vi "V004 - Final Labview.vi"() -> ()   [LabVIEW 2022 SP3]
uses:
  <vilib>/DAQmx/read.llb/DAQmx Read (Analog 1D DBL NChan 1Samp).vi
  <vilib>/DAQmx/create/channels.llb/DAQmx Create Channel (AI-Voltage-Basic).vi
  <vilib>/DAQmx/miscellaneous.llb/DAQmx Fill In Error Info.vi
panel:
  out "High Temperature":bool
  out "High Humidity":bool
  out "Fan Speed Chart":dbl(graph)
  out "Humidity Chart":dbl(graph)
  out "Temperature Chart":dbl(graph)
  in  "Turn Off":bool
  out "Speed 3":bool
  out "Humidity":dbl(knob) scale=0.0..100.0
  out "Temperature":dbl(knob) scale=0.0..40.0
  out "Speed 2":bool
  out "Speed 1":bool
  in  "Numeric Controller Sub":dbl format="%#_1g"
  out "Power On":bool
  in  "Power On":bool
  out "Connected":bool
  in  "VISA resource name":refnum<visa-resource-name>
  in  "Connect":bool
  in  "Numeric Controller Main":dbl
  # "SMART FAN"
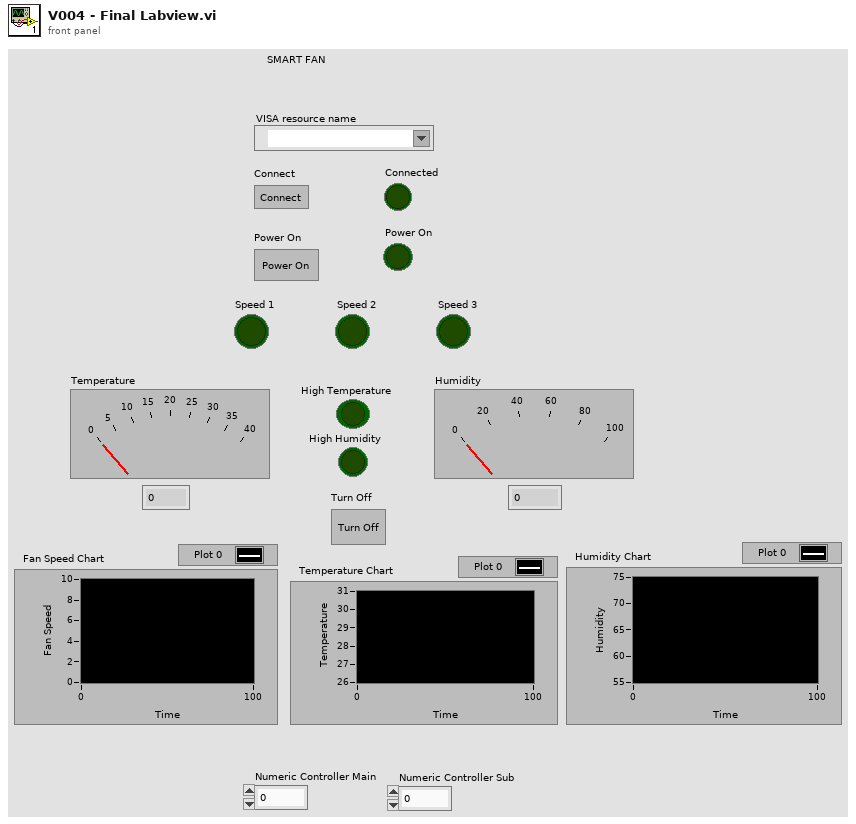
[diagram p1: front panel]
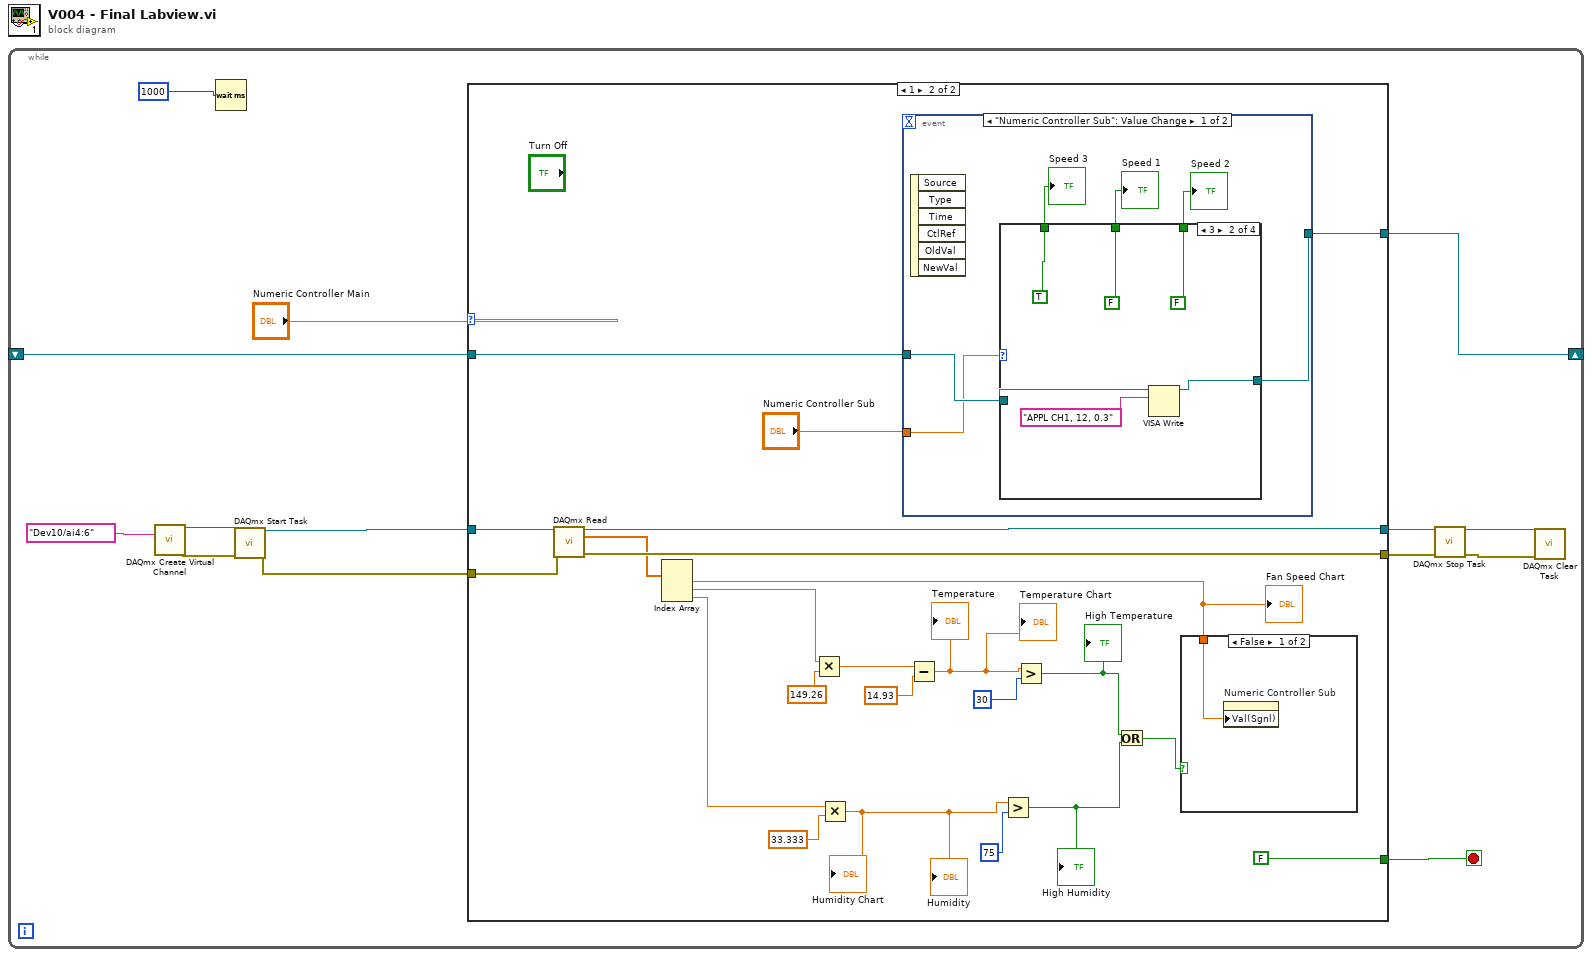
[diagram p0: block diagram]
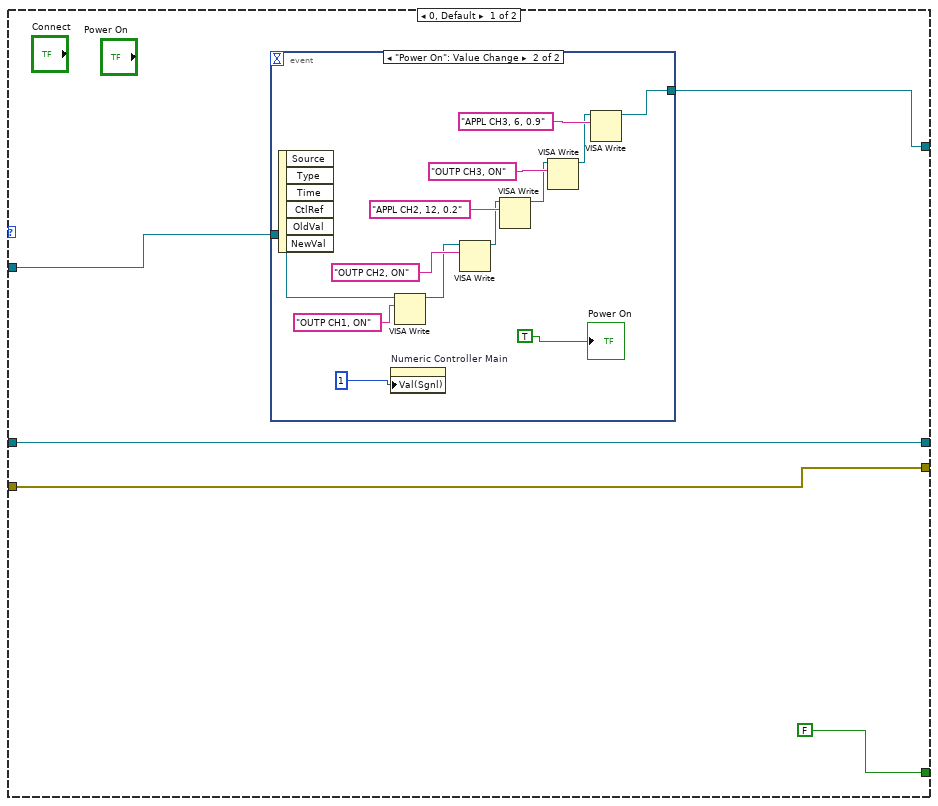
[diagram p2: hidden frame]
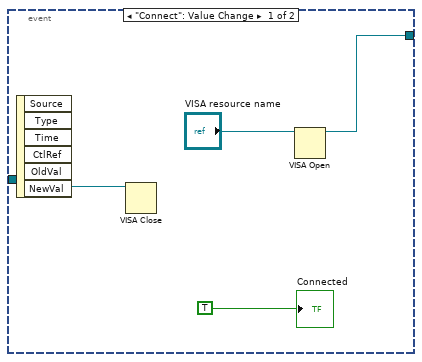
[diagram p3: hidden frame]
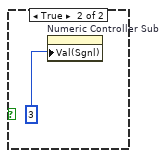
[diagram p4: hidden frame]
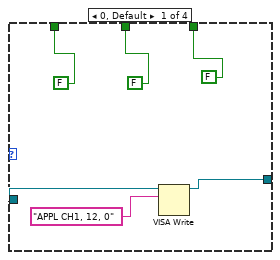
[diagram p5: hidden frame]
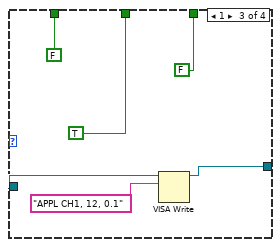
[diagram p6: hidden frame]
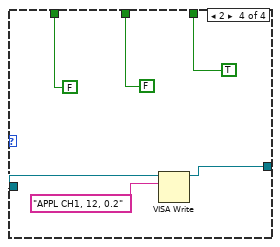
[diagram p7: hidden frame]
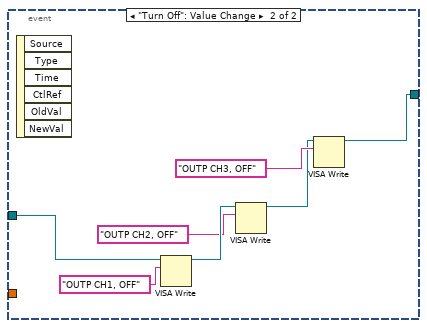
[diagram p8: hidden frame]
diagram:
  n1 = while {
    shift-right: [w13] -> _
    shift-left: _ -> [w14]
    stop <- w12 stop-if-true
    n2 = call-poly <vilib>:"DAQmx Create Virtual Channel.vi"("physical channels"=tag "Dev10/ai4:6") -> ("task out"=w10:refnum<k21>, "error out"=w6:errorcluster)  [unwired: 13 in]
    n3 = Wait (ms)(milliseconds to wait=1000) -> ()  [unwired: 1 out]
    n4 = call <vilib>:"DAQmx Start Task.vi"("task/channels in"=w10, "error in"=w6) -> ("task out"=w8:refnum<k21>, "error out"=w7:errorcluster)  [unwired: 12 in]
    n5 = case shown="1" "Numeric Controller Main" {
      tunnel: w14 -> [w19 w57]
      tunnel: [w18 w58] -> w13
      tunnel: [FALSE FALSE] -> w12
      tunnel: w8 -> [w16 w55]
      tunnel: w7 -> [w15 w54]
      tunnel: [w16 w53] -> w2
      tunnel: [w15 w52] -> w1
      frame 0, Default {
        n6 = event shown="[1] \"Power On\": Value Change" {
          selector: _ -> [_ _]
          dyn-events: _ -> [_ _]
          timeout: _ -> [_ _]
          tunnel: w19 -> [w23 w35]
          tunnel: [w22 w25] -> w18
          event "Connect": Value Change {
            n7 = event-data() -> ()  [unwired: 1 in, 6 out]
            n8 = VISA Close(VISA resource name=w23) -> ()  [unwired: 1 in, 1 out]
            n9 = VISA Open(VISA resource name="VISA resource name") -> (VISA resource name=w22:refnum<visa-resource-name>)  [unwired: 4 in, 1 out]
            "Connected" <- TRUE
          }
          event "Power On": Value Change {
            n10 = event-data() -> ()  [unwired: 1 in, 6 out]
            n11 = property on="Numeric Controller Main" class="DigNum (strict)"("Val(Sgnl)"=1) -> ()  [unwired: 2 in, 2 out]
            n12 = VISA Write(VISA resource name=w35, write buffer="OUTP CH1, ON") -> (VISA resource name out=w32:refnum<visa-resource-name>)  [unwired: 1 in, 2 out]
            n13 = VISA Write(VISA resource name=w32, write buffer="OUTP CH2, ON") -> (VISA resource name out=w30:refnum<visa-resource-name>)  [unwired: 1 in, 2 out]
            n14 = VISA Write(VISA resource name=w30, write buffer="APPL CH2, 12, 0.2") -> (VISA resource name out=w28:refnum<visa-resource-name>)  [unwired: 1 in, 2 out]
            n15 = VISA Write(VISA resource name=w28, write buffer="OUTP CH3, ON") -> (VISA resource name out=w26:refnum<visa-resource-name>)  [unwired: 1 in, 2 out]
            n16 = VISA Write(VISA resource name=w26, write buffer="APPL CH3, 6, 0.9") -> (VISA resource name out=w25:refnum<visa-resource-name>)  [unwired: 1 in, 2 out]
            "Power On" <- TRUE
          }
        }
      }
      frame 1 {
        n17 = call-poly <vilib>:"DAQmx Read.vi"("task/channels in"=w55, "error in"=w54) -> ("task out"=w53:refnum<k21>, "data"=w51:dbl[], "error out"=w52:errorcluster)  [unwired: 11 in]
        n18 = Index Array(array=w51) -> (element #1=w37:dbl, element #2=w47:dbl, element #3=w46:dbl)  [unwired: 3 in]
        "Fan Speed Chart" <- w37
        n19 = Multiply(x=w47, y=149.26) -> (x*y=w49:dbl)
        n20 = Multiply(x=w46, y=33.333) -> (x*y=w38:dbl)
        "Humidity" <- w38
        "Humidity Chart" <- w38
        n21 = event shown="[0] \"Numeric Controller Sub\": Value Change" {
          selector: _ -> [_ _]
          dyn-events: _ -> [_ _]
          timeout: _ -> [_ _]
          tunnel: [w67 w92] -> w58
          tunnel: w57 -> [w66 w97]
          tunnel: "Numeric Controller Sub" -> [w65 _]
          event "Numeric Controller Sub": Value Change {
            n22 = event-data() -> ()  [unwired: 1 in, 6 out]
            n23 = case shown="3" w65 {
              tunnel: [w72 w78 w84 w90] -> w67
              tunnel: w66 -> [w71 w77 w83 w89]
              tunnel: [FALSE TRUE FALSE FALSE] -> w64
              tunnel: [FALSE FALSE TRUE FALSE] -> w63
              tunnel: [FALSE FALSE FALSE TRUE] -> w62
              frame 0, Default {
                n24 = VISA Write(VISA resource name=w71, write buffer="APPL CH1, 12, 0") -> (VISA resource name out=w72:refnum<visa-resource-name>)  [unwired: 1 in, 2 out]
              }
              frame 3 {
                n25 = VISA Write(VISA resource name=w77, write buffer="APPL CH1, 12, 0.3") -> (VISA resource name out=w78:refnum<visa-resource-name>)  [unwired: 1 in, 2 out]
              }
              frame 1 {
                n26 = VISA Write(VISA resource name=w83, write buffer="APPL CH1, 12, 0.1") -> (VISA resource name out=w84:refnum<visa-resource-name>)  [unwired: 1 in, 2 out]
              }
              frame 2 {
                n27 = VISA Write(VISA resource name=w89, write buffer="APPL CH1, 12, 0.2") -> (VISA resource name out=w90:refnum<visa-resource-name>)  [unwired: 1 in, 2 out]
              }
            }
            "Speed 3" <- w64
            "Speed 1" <- w63
            "Speed 2" <- w62
          }
          event "Turn Off": Value Change {
            n28 = event-data() -> ()  [unwired: 1 in, 6 out]
            n29 = VISA Write(VISA resource name=w97, write buffer="OUTP CH1, OFF") -> (VISA resource name out=w96:refnum<visa-resource-name>)  [unwired: 1 in, 2 out]
            n30 = VISA Write(VISA resource name=w96, write buffer="OUTP CH2, OFF") -> (VISA resource name out=w93:refnum<visa-resource-name>)  [unwired: 1 in, 2 out]
            n31 = VISA Write(VISA resource name=w93, write buffer="OUTP CH3, OFF") -> (VISA resource name out=w92:refnum<visa-resource-name>)  [unwired: 1 in, 2 out]
          }
        }
        n32 = Subtract(x=w49, y=14.93) -> (x-y=w39:dbl)
        "Temperature" <- w39
        "Temperature Chart" <- w39
        n33 = Greater?(x=w38, y=75) -> (0:w41:bool)
        "High Humidity" <- w41
        n34 = Greater?(x=w39, y=30) -> (0:w42:bool)
        "High Temperature" <- w42
        n35 = Or(x=w42, y=w41) -> (x .or. y?=w40:bool)
        n36 = case shown="False" w40 {
          tunnel: w37 -> [w60 _]
          frame False {
            n37 = property on="Numeric Controller Sub" class="DigNum (strict)"("Val(Sgnl)"=w60) -> ()  [unwired: 2 in, 2 out]
          }
          frame True {
            n38 = property on="Numeric Controller Sub" class="DigNum (strict)"("Val(Sgnl)"=3) -> ()  [unwired: 2 in, 2 out]
          }
        }
      }
    }
    n39 = call <vilib>:"DAQmx Stop Task.vi"("task/channels in"=w2, "error in"=w1) -> ("task out"=w4:refnum<k21>, "error out"=w3:errorcluster)  [unwired: 12 in]
    n40 = call <vilib>:"DAQmx Clear Task.vi"("task in"=w4, "error in"=w3) -> ()  [unwired: 13 in, 1 out]
  }
